vi "AlliGator Run Source Image Python Function.vi"(8 "error in (no error)":errorcluster, 9 "Source Image":T5, 10 "Python Function Info":T1={"Script Path"=path "", "Function Name"="", "Function Parent Menu"="", "Function Input Parameters"=[], "Function Outputs"=[], "Function Doc String"="", "Function Display Name"="", "Function Target Type"=enum."Window Menu", "Function Target Window"="", "Parent Menu Location"="", "Item Menu Tag"="", "Is preceded by Separator"=FALSE}, 11 "Data Value Reference in":refnum<data-value>) -> (0 "error out":errorcluster, 1 "Message":string, 2 "Function Output Type":string, 3 "Data Value Reference out":refnum<data-value>)   [LabVIEW 2021, in "AlliGator Python Plugins.lvlib"]
doc: "Runs image-related python function."
uses:
  AlliGator Python Plugins.lvlib
  AlliGator Internal Variables v2.ctl
  <vilib>/vision/Image Controls.llb/IMAQ Image.ctl
  AlliGator Gate Image Set.ctl
  AlliGator FLI Dataset Type.ctl
  AlliGator Data Series Type.ctl
  AlliGator Dataset Channel.ctl
  AlliGator Gate Arithmetic.ctl
  AlliGator Displayed Image.ctl
  Image/Named ROI Description.ctl
  AlliGator Decay Metadata v3.ctl
  AlliGator Decay Background Subtraction Info.ctl
  AlliGator Baseline Subtraction Method.ctl
  Graphs/XY Graph/XY Graph Plot Shift Parameters.ctl
  Graphs/XY Graph/XY Graph Plot Shift Method.ctl
  AlliGator Decay Extrapolation Parameters.ctl
  Phasor/Calibration Phasor (m, phi).ctl
  Phasor/Phasor Reference Series.ctl
  Phasor/Phasor Calibration Map v2.ctl
  Phasor/Phasor (g, s).ctl
  AlliGator Raw Phasor Plot Data v4.ctl
  Phasor/Phasor Standard Deviation Options.ctl
  AlliGator Phasor Multi-Harmonic Data.ctl
  Phasor/Phasor Harmonic Data.ctl
  AlliGator Decay Fit Options & Parameters v2.ctl
  Fits/IRF(X)PSED/Decay Fit Options v2.ctl
  Fits/Decay Convolution/Decay Model.ctl
  Fits/Residual Type.ctl
  Fits/IRF(X)PSED/Fit Weights Type.ctl
  Fits/Non-linear Fitting Method v2.ctl
  Fits/Fit Calculation Method.ctl
  Fits/Non-linear Fitting Algorithm.ctl
  AlliGator Decay Fit Parameter Constraints 2.ctl
  Fits/IRF(X)PSED/Decay Fit Parameters In List.ctl
  Fits/IRF(X)PSED/MLE Baseline Offset Type.ctl
  AlliGator Decay Preprocessing Parameters.ctl
  Fits/IRF(X)PSED/Decay Fit Parameters & Derived Quantities List.ctl
  AlliGator Python Function Information.ctl
  AlliGator Python Function Parameter Definition.ctl
  AlliGator Python Function Output Definition.ctl
  AlliGator Python Plugin Target Type.ctl
  AlliGator Variables List.ctl
  AlliGator Python Plugin Image Data.ctl
  AlliGator Globals, Variables & Constants.lvlib
  AlliGator Source Image.lvlib
  Error/Error.lvlib
  Phasor/Phasor.lvlib
  Image/Image.lvlib
  AlliGator Decay Preprocessing.lvlib
  Graphs/XY Graph/XY Graph Add-Ons.lvlib
  AlliGator Phasor Graph.lvlib
  AlliGator Files.lvlib
  AlliGator Phasor Plot.lvlib
  Fits/Fits.lvlib
  AlliGator Decay Fit.lvlib
  AlliGator Decay Fit Parameter Map.lvlib
  AlliGator Internal Variables.lvlib
  AlliGator Settings.lvlib
  AlliGator Dual-Channel Datasets.lvlib
panel:
  out "session out":refnum<k35>
  out "Function Parameters String":string
  # "see the AlliGator License on the block diagram (Ctrl+E or Window:Show Block Diagram)"
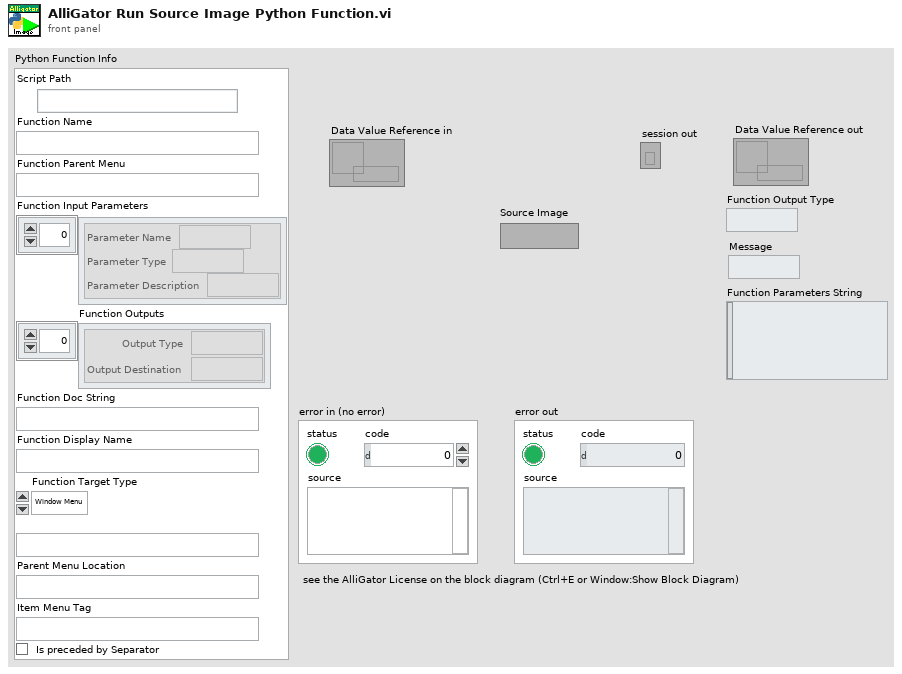
[diagram p1: front panel]
types:
  T1 = typedef "AlliGator Python Plugins.lvlib/AlliGator Python Function Information.ctl" = cluster{"Script Path":path, "Function Name":string, "Function Parent Menu":string, "Function Input Parameters":T2[], "Function Outputs":T3[], "Function Doc String":string, "Function Display Name":string, "Function Target Type":T4, "Function Target Window":string, "Parent Menu Location":string, "Item Menu Tag":string, "Is preceded by Separator":bool}
  T2 = typedef "AlliGator Python Plugins.lvlib/AlliGator Python Function Parameter Definition.ctl" = cluster{"Parameter Name":string, "Parameter Type":string, "Parameter Description":string}
  T3 = typedef "AlliGator Python Plugins.lvlib/AlliGator Python Function Output Definition.ctl" = cluster{"Output Type":string, "Output Destination":string}
  T4 = typedef "AlliGator Python Plugins.lvlib/AlliGator Python Plugin Target Type.ctl" = enum16{"Undefined", "Window Menu", "Object Menu"}
  T5 = typedef "IMAQ Image.ctl" = refnum<image>
  T6 = typedef "AlliGator Python Plugins.lvlib/AlliGator Python Plugin Image Data.ctl" = cluster{"Image_Name":string, "Image":sgl[][]}
  T7 = typedef "AlliGator Source Image.lvlib/AlliGator Displayed Image.ctl" = enum16{"Single Gate", "Sum of All Gates", "Max of All Gates", "Min of All Gates", "-", "White Ligth Image", "Mask Image"}
  T8 = typedef "AlliGator Globals, Variables & Constants.lvlib/AlliGator Variables List.ctl" = enum16{"---- GUI ----", "Initialization Status", "State Indicators Refnum", "Original AlliGator Menu Items", "Current Action Loop State", "Script in progress", "Playback", "Loop Playback", "Search ROI Used", "Search ROI", "Decay Graph Max Legend Size", "Intensity Graph Max Legend Size", "Decay Statistics Graph Max Legend Size", "Phasor Graph Max Legend Size", "Phasor Ratio Graph Max Legend Size", "Lifetime Graph Max Legend Size", "---- Files ----", "Export Dataset Frames as Individual Files", "Show Batch Export Help Balloons", "Frames in Dataset", "ptu File Frame Start Indices", "Current Frame in Dataset", "Current Frame Timestamp", "------ Python Plugins ------", "Python Plugins Information", "Python Session", "Valid Python Session?", "---- Source Image ----", "Dataset Loaded", "Dataset Metadata", "Dataset Channel", "Dataset Data Description", "Background Dataset Metadata", "Background Dataset Channel", "Background Dataset Data Description", "Background File Subtraction", "Background File Path", "Background File Pile-up Correction", "Background File Pixel Well Capacity", "Background File Scaling Factor", "Source Image ROIs", "Current Source Image ROI", "Source Image ROI Event Refnum", "X_Source Image Display Range", "X_Source Image Palette Information", "Source Image Palette List", "Source Image Scale", "Current Dataset Load Settings", "Source Image:ROI Overlay Color", "---- Image Profile Window ----", "Image Profile:Overlay ROI in Source Image", "Image Profile Window Event Refnum", "Image Profile:IntensityType", "Image Profile:Intensity Average Type", "Image Profile:Intensity-weighted SDV", "Image Profile:Box Profile Type", "Image Profile Window Open", "Image Profile:Plotted Fit Parameter", "X_Type of Displayed Image", "X_Time Gate Slider", "Dataset Path", "Source Image Overlay to Erase", "Is Displayed Image Accumulated", "White Light Image Modified", "Mask Image Modified", "Macrotime Gate Separation", "------ Phasor Graph -------", "Phasor Graph:Show Line", "---- Phasor Plot ---", "Phasor Plot Parameters Changed", "FLI Dataset Modified since last Phasor Plot Calculation", "Phasor Harmonics Data", "Selected Phasor Harmonics", "Phasor Harmonic Manager Event Refnum", "Phasor Plot ROIs", "Current Phasor Plot ROI", "Phasor Plot ROI Event Refnum", "Phasor Plot Image Reference Points", "Phasor Plot Computed", "Phasor Plot Palette Information", "Phasor Plot Palette List", "Phasor Ratio Palette Information", "Phasor Ratio Palette List", "Phasor Image Scale", "Phasor Plot Image Overlay to Erase", "Phasor Plot Image Elements to Update", "Current Phasor Plot Calculation Parameters", "Current Phasor Calibration Options", "Reset Cumulated Phasor Plot", "Phasor Ratio Reference 1", "Phasor Ratio Lifetime Reference 1", "Phasor Ratio Reference 1 Frequency", "Phasor Ratio Reference 2", "Phasor Ratio Lifetime Reference 2", "Phasor Ratio Reference 2 Frequency", "---- Decay Analysis ----", "Number of Selected Decays to Fit", "LS Fit Results", "LAR Fit Results", "BS Fit Results", "Last Decay Max - Min", "Best Fit Parameters", "Best Fit Parameter Names", "Actual Size X", "Actual Size Y", "Binning X", "Binning Y", "Actual # Gates", "Dataset Number", "Gates to...", "Gates Skipped", "Gates to keep", "Gate Step", "Gate Separation", "Reversed Gates", "Pile-up Correction", "Pixel Well Capacity", "Background Subtracted", "Background Subtraction Method", "Background Definition Range", "Background File (deprecated)", "Number of Dataset Accumulated", "Array of Accumulated Dataset Paths", "Do Averaged Datasets", "Destination File Path", "Process Plot Target", "Use 1/D as Phasor Frequency", "---- Decay Fit Parameter Map -----", "Decay Fit Parameter Map Palette Information", "Decay Fit Parameter Map Palette List", "Local Decay Graph Window Event Refnum", "------- Local Decay Window ---------", "Use normalized IRF for convolution", "----- Miscellaneous ----", "Skippable Dialog Windows Status"}
  T9 = typedef "AlliGator Internal Variables.lvlib/AlliGator Internal Variables v2.ctl" = cluster{"Displayed Image":T5, "White Light Image":T5, "Mask Image":T5, "ROI Mask Image":T5, "Current Dataset Images 1":T10, "Background Dataset Images 1":T10, "Current Dataset Images 2":T10, "Background Dataset Images 2":T10, "Current Dataset Arithmetic Images":T10, "Accumulated Dataset Images 1":T10, "Accumulated Dataset Images 2":T10, "Accumulated Dataset Arithmetic Images":T10, "Phasor Plot Image":T5, "Decay Fit Parameter Map Image":T5, "Single Data Point Path":path, "White Light Image Path":path, "Mask Image Path":path, "Time-Series Folder":path, "[Time-Series Paths]":path[], "Current Dataset":i32, "Single Dataset Type":T11, "Current Folder":string, "AlliGator Data Series Type":T12, "# Datasets":i32, "Dual-Channel Dataset":bool, "Selected Channel Name":string, "Dataset Channel":T13, "Channel Arithmetic":T14, "Dual-Channel Background Dataset":bool, "Background Channel":T13, "Dual-Channel Accumulated Dataset":bool, "Start Time":dbl, "[Time-Series Timestamps]":dbl[], "[Intensity Corrections]":dbl[], "Time Series Script":bool, "Type of Displayed Image":T7, "Gate Image Slide":u16, "# Gates":i32, "ROIs":T15[], "ROI Decay":cluster{"t Array":dbl[], "I Array":dbl[]}, "Valid Decay":bool, "Decay  Metadata":T17, "Reference Decay Plot Name":string, "Reference Decay":cluster{"t Array":dbl[], "I Array":dbl[]}, "Decay Shift Plot":cluster{"Time Stamps":dbl[], "Decay Shifts":dbl[]}, "[Decays Max Values]":sgl[], "[Decays Min Values]":sgl[], "Calibration Phasor":T23, "Calibration Phasor Series":T24, "Phasor Calibration Map":T25, "Calibration Map MD5 Digest":string, "Last Raw Phasor":T26, "Last Calibrated Phasor":T26, "Last Calibrated Phasor SDV":T26, "Phasor Graph:Phasor Plot":cluster{"g Array":dbl[], "s Array":dbl[]}, "Phasor Graph:Phasor SDV Plot":cluster{"g Array":dbl[], "s Array":dbl[]}, "[Phasor Graph:Raw Phasor Plots]":T27[], "Phasor Plot locked to Ref 1":i32, "[Phasor Plot(s) locked to Ref 1]":i32[], "[Phasor Plot(s) locked to Ref 2]":i32[], "[Pixel Phasors]":T26[], "[[Sum Image]]":dbl[][], "[[CSG Phasors]]":csg[][], "[[Valid Pixel?]]":bool[][], "I/m/phi Dataset":cluster{"I/m/phi Dataset?":bool, "Base Frequency":dbl[unit], "Harmonic Orders":u8[]}, "Multi Phasor Plot Data":T29, "Decay Fit Options & Parameters":T31, "Fit Options: Decay Preprocessing Parameters":T42, "Fit Options: Reference Decay":cluster{"t Array":dbl[], "I Array":dbl[]}, "Is Full Image Parameters Map":bool, "Is Single-Pixels Parameters Map":bool, "NLSF Parameters Map X Resolution":i32, "NLSF Parameters Map Y Resolution":i32, "[Single Decay Fit Parameters]":dbl[], "Fit Model":T33, "[[Multiple Decays Fit Parameters]]":dbl[][], "[[Multiple Decays Fit Parameter SDVs]]":dbl[][], "[[IRFs]]":dbl[][], "IRF Array Time Axis":dbl[], "Decay Array Time Axis":dbl[], "[Decay Fit Parameter Names]":T43[], "[[Phasor Ratios]]":dbl[][], "[[Average Lifetimes]]":dbl[][], "Amplitude Weighted Average Lifetime":bool, "[Decay Sum]":dbl[], "[[User-defined Quantities]]":dbl[][], "User-defined Quantity":string}
  T10 = typedef "AlliGator Internal Variables.lvlib/AlliGator Gate Image Set.ctl" = cluster{"SGL Image Max":T5, "SGL Image Sum":T5, "SGL Gate Images":T5[], "SGL Image Min":T5}
  T11 = typedef "AlliGator Files.lvlib/AlliGator FLI Dataset Type.ctl" = enum16{"HDF5 FLI Dataset", "Gate Image Folder", ".sdt FLI Dataset (Becker & Hickl)", ".ptu FLI Dataset (PicoQuant)", "SS1 FLI Dataset", "SS2 FLI Dataset", "I/m/phi Dataset", ".bin FLI Dataset (PicoQuant Binned)", ".bin FLI Dataset (Piccolo Binned)"}
  T12 = typedef "AlliGator Files.lvlib/AlliGator Data Series Type.ctl" = enum16{"Not a Supported Series", "Gate Images Folder Series", "SwissSPAD 2 Dataset Series", "B&H FLI Dataset Series", "PicoQuant PTU FLI Dataset Series", "PicoQuant BIN FLI Dataset Series", "Piccolo hist BIN FLI Dataset Series", "HDF5 FLI Dataset Series"}
  T13 = typedef "AlliGator Dual-Channel Datasets.lvlib/AlliGator Dataset Channel.ctl" = enum16{"G2", "INT"}
  T14 = typedef "AlliGator Settings.lvlib/AlliGator Gate Arithmetic.ctl" = enum16{"None", "INT-G2", "G2/INT*<INT>", "(1 - G2/INT)*<INT>"}
  T15 = typedef "Image.lvlib/Named ROI Description.ctl" = cluster{"ROI Descriptor":T16, "ROI Name":string, "Overlay Color":u32}
  T16 = typedef "ROI Descriptor" = cluster{"Global Rectangle":i32[], "Contours":cluster{"ID":enum32{"External", "Internal"}, "Type":u32, "Coordinates":i32[]}[]}
  T17 = typedef "AlliGator Phasor Graph.lvlib/AlliGator Decay Metadata v3.ctl" = cluster{"ROI Descriptor":T16, "ROI Center":cluster{"X":i32, "Y":i32}, "Decay Background Subtraction Info":T18, "Decay Reverted":bool, "Decay Smoothened":bool, "Decay Straightened":bool, "Fitted Tau (Decay Straightening)":dbl, "Decay Shift Parameters":T20, "Decay Shifted":bool, "Decay Extrapolated":bool, "Decay Extrapolation Parameters":T22, "Decay Normalized":bool, "Fold Decay":bool, "# Folds":u32}
  T18 = typedef "AlliGator Decay Analysis.lvlib/AlliGator Decay Preprocessing.lvlib/AlliGator Decay Background Subtraction Info.ctl" = cluster{"Laser Period":dbl[unit], "Gate Duration":dbl[unit], "Baseline Subtraction Method":T19, "Background Definition Range":cluster{"Min Gate":dbl[unit], "Max Gate":dbl[unit]}, "Total Intensity w/o Bkgd Subtraction":dbl, "Bkgd-subtracted Intensity (exp)":dbl, "# Data Points":i32, "Background/Gate":dbl, "Fitted Lifetime":dbl[unit], "Bkgd-subtracted Intensity (theo)":dbl}
  T19 = typedef "AlliGator Decay Analysis.lvlib/AlliGator Decay Preprocessing.lvlib/AlliGator Baseline Subtraction Method.ctl" = enum16{"Mean", "Min", "Square Gated Single-Exponential", "File", "Constant"}
  T20 = typedef "XY Graph Add-Ons.lvlib/XY Graph Plot Shift Parameters.ctl" = cluster{"Type":T21, "Shift":dbl[unit], "Threshold":dbl, "Rotate":bool}
  T21 = typedef "XY Graph Add-Ons.lvlib/XY Graph Plot Shift Method.ctl" = enum16{"Default", "CFD", "Threshold", "Cross-Correlation"}
  T22 = typedef "AlliGator Decay Analysis.lvlib/AlliGator Decay Preprocessing.lvlib/AlliGator Decay Extrapolation Parameters.ctl" = cluster{"Additional Points":u32, "Head Fraction":dbl, "Fitted Tau":dbl, "Use Periodicity":bool, "Use Cursors":bool, "Tail Fraction":dbl}
  T23 = typedef "Phasor.lvlib/Calibration Phasor (m, phi).ctl" = cluster{"m":dbl, "phi":dbl, "Phasor Frequency":dbl[unit], "Reference Lifetime":dbl[unit]}
  T24 = typedef "Phasor.lvlib/Phasor Reference Series.ctl" = cluster{"m Array":dbl[], "phi Array":dbl[], "Phasor Frequency":dbl[unit], "Calibration Lifetime":dbl[unit]}
  T25 = typedef "Phasor.lvlib/Phasor Calibration Map v2.ctl" = cluster{"Phasor Frequency":dbl[unit], "Calibration Lifetime":dbl[unit], "ROI Centers":cluster{"X":i32, "Y":i32}[], "ROI Descriptors":T16[], "Map Resolution X":i32, "Map Resolution Y":i32, "z Array":cdb[]}
  T26 = typedef "Phasor.lvlib/Phasor (g, s).ctl" = cluster{"g":dbl, "s":dbl}
  T27 = typedef "AlliGator Phasor Graph.lvlib/AlliGator Raw Phasor Plot Data v4.ctl" = cluster{"Phasor Plot Name":string, "Raw Phasor Plot":T26[], "Phasor Frequency":dbl[unit], "[Decay Metadata]":T17[], "Raw Phasor Plot SDV":T26[], "Phasor SDV Options":T28, "[Calibration Phasor]":T23[]}
  T28 = typedef "Phasor.lvlib/Phasor Standard Deviation Options.ctl" = cluster{"Compute Estimated SDV":bool, "# Replicas":u32, "Use Estimated Average Phasor":bool}
  T29 = typedef "AlliGator Phasor Plot.lvlib/AlliGator Phasor Multi-Harmonic Data.ctl" = cluster{"Base Frequency":dbl[unit], "# Harmonics":u8, "Harmonic Orders":u8[], "Phasor Plot Settings Checksum":u64, "Phasor Harmonic Data Array":T30[]}
  T30 = typedef "Phasor.lvlib/Phasor Harmonic Data.ctl" = cluster{"Phasor Harmonic Name":string, "Phasor Plot Settings Checksum":u64, "Phasor Frequency":dbl[unit], "Base Frequency":dbl[unit], "Harmonic Order":u8, "Phasor Plot Parameters":string, "Phasor Array [[CSG]]":csg[][], "Dataset File Path":path}
  T31 = typedef "AlliGator Decay Fit Parameter Map.lvlib/AlliGator Decay Fit Options & Parameters v2.ctl" = cluster{"SYNC Period":dbl[unit], "Fit Options":T32, "Fit Parameter Constraints":T39[], "MLE Baseline Offset":dbl, "MLE Baseline Offset Type":T41}
  T32 = typedef "Fits.lvlib/Decay Fit Options v2.ctl" = cluster{"Show Fit Residuals":bool, "Fit Model":T33, "Residual Type":T34, "Max Decay Percentile":dbl, "Min Decay Percentile":dbl, "Show Full Decay":bool, "Weights":T35, "Fitting Method":T36, "Compute Parameter Uncertainties":bool, "Periodic Boundaries":bool, "Model Calculation":T37, "Period":dbl[unit], "Termination Criteria":cluster{"Max Iterations":i32, "Max Function Calls":i32, "Max Time":dbl[unit], "Function Tolerance":dbl, "Parameter Tolerance":dbl, "Gradient Tolerance":dbl, "Min Lambda":dbl, "Max Lambda":dbl, "Initial Tick Count":u32}, "Offset Resolution":dbl[unit], "Use Local IRF":bool, "Fitting Algorithm":T38}
  T33 = typedef "Fits.lvlib/Decay Model.ctl" = enum16{"1-Exponential", "2-Exponentials"}
  T34 = typedef "Fits.lvlib/Residual Type.ctl" = enum16{"Standard", "Normalized", "Reduced"}
  T35 = typedef "Fits.lvlib/Fit Weights Type.ctl" = enum16{"Unweighted", "1/Variance", "Best of All"}
  T36 = typedef "Fits.lvlib/Non-linear Fitting Method v2.ctl" = enum16{"Least Square", "Least Absolute Residual", "Bisquare", "MLE", "-", "Best of All"}
  T37 = typedef "Fits.lvlib/Fit Calculation Method.ctl" = enum16{"Simulation", "Convolution", "Integration"}
  T38 = typedef "Fits.lvlib/Non-linear Fitting Algorithm.ctl" = enum16{"Levenberg-Marquardt", "Trust-Region Dogleg"}
  T39 = typedef "AlliGator Decay Analysis.lvlib/AlliGator Decay Fit.lvlib/AlliGator Decay Fit Parameter Constraints 2.ctl" = cluster{"Fit Parameter":T40, "Min Value":dbl, "Max Value":dbl, "Global":bool, "Used":bool}
  T40 = typedef "Fits.lvlib/Decay Fit Parameters In List.ctl" = enum16{"Offset", "Baseline", "A_1", "tau_1", "A_2", "tau_2"}
  T41 = typedef "Fits.lvlib/MLE Baseline Offset Type.ctl" = enum32{"Absolute", "Percentage"}
  T42 = typedef "AlliGator Decay Analysis.lvlib/AlliGator Decay Preprocessing.lvlib/AlliGator Decay Preprocessing Parameters.ctl" = cluster{"Background Subtraction":bool, "Straighten Decay":bool, "Reverse Gates":bool, "1-Normalized Decay":bool, "Smoothen Decay":bool, "Smoothing Parameter":dbl, "Shift Decay":bool, "Decay Shift Parameters":T20, "Extrapolate Decay":bool, "Additional Points":u32, "Head Fraction":dbl, "Pixel-Normalize Decay":bool, "Use Periodicity":bool, "Use Cursors":bool, "Tail Fraction":dbl, "Use Decay Pre-Processing":bool, "Fold Decay":bool, "# Folds":u32, "[0-1]-Normalized Decay":bool}
  T43 = typedef "Fits.lvlib/Decay Fit Parameters & Derived Quantities List.ctl" = enum16{"Offset", "Baseline", "A_1", "tau_1", "A_2", "tau_2", "<tau>_a", "f1_a", "f2_a", "<tau>_i", "f1_i", "f2_i", "-", "R^2", "Chi^2"}
  T44 = typedef "Image Type" = u32
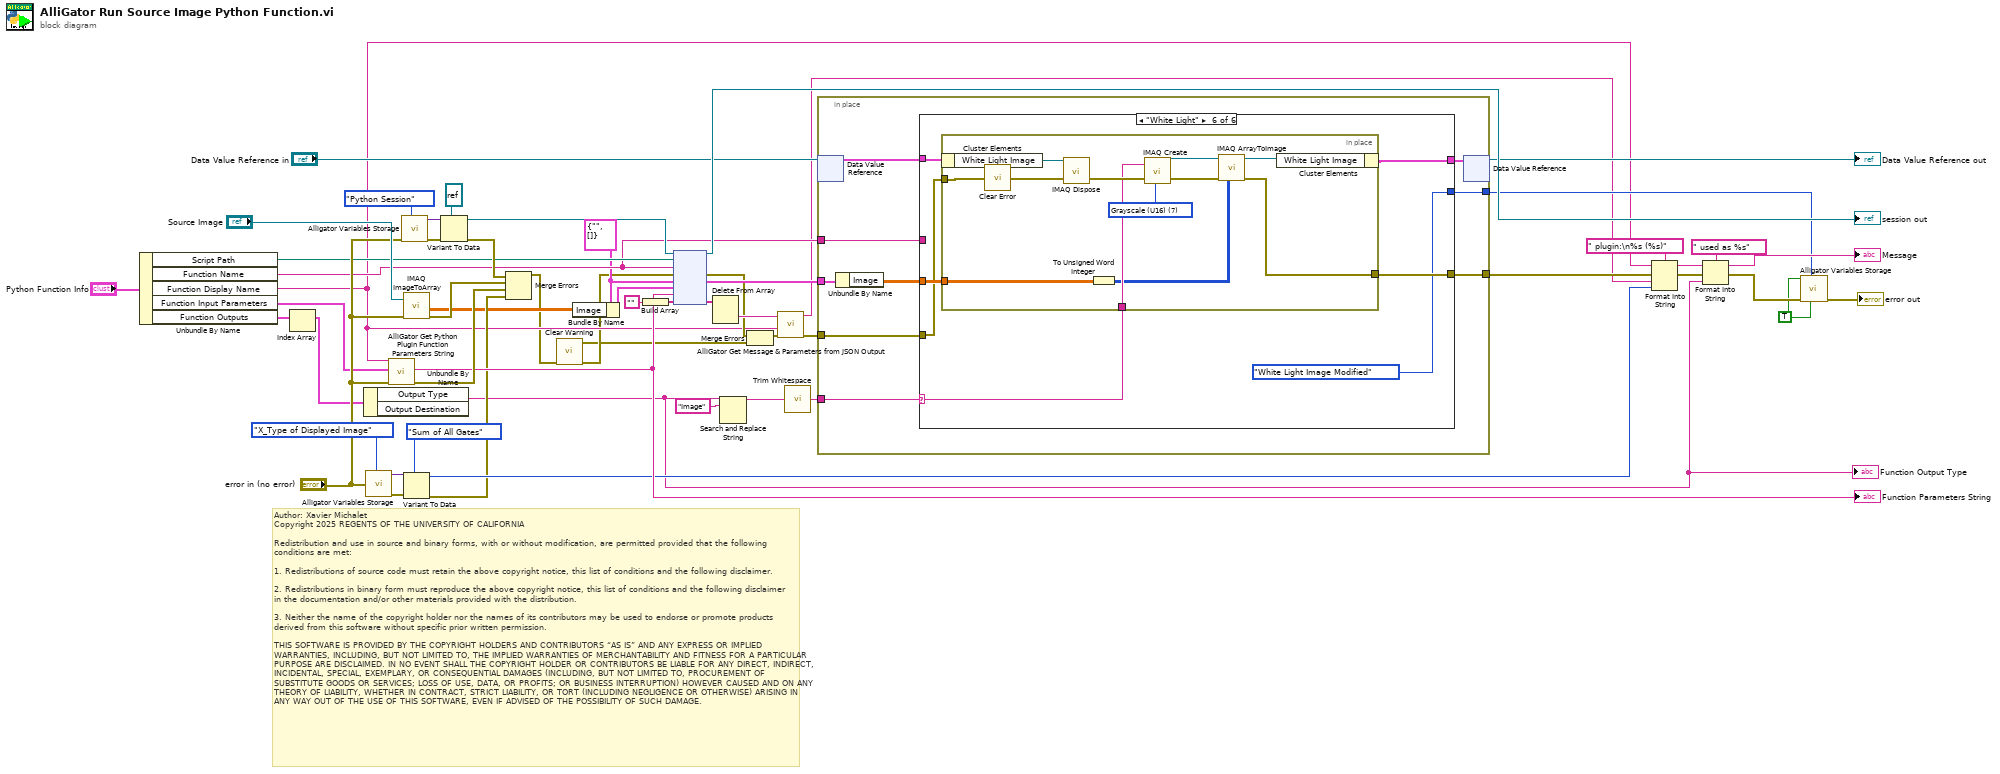
[diagram p0: block diagram]
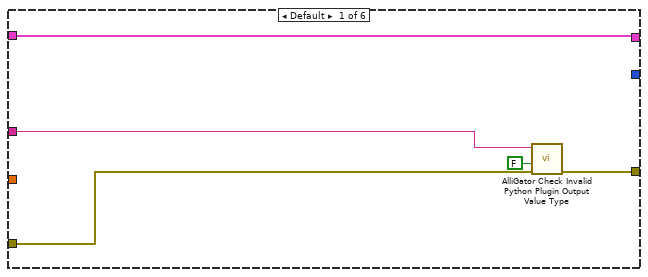
[diagram p2: hidden frame]
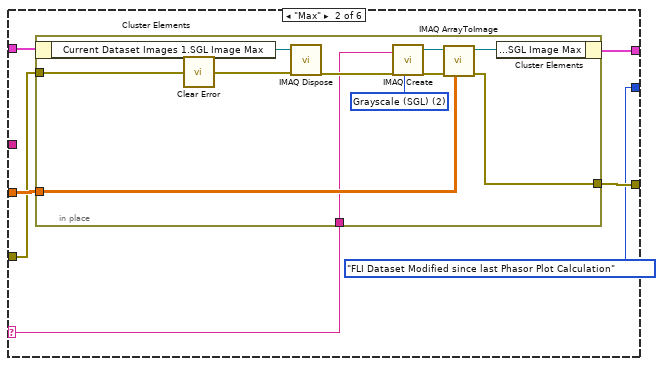
[diagram p3: hidden frame]
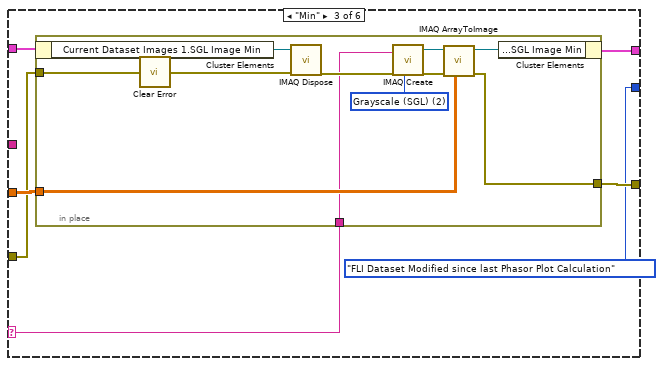
[diagram p4: hidden frame]
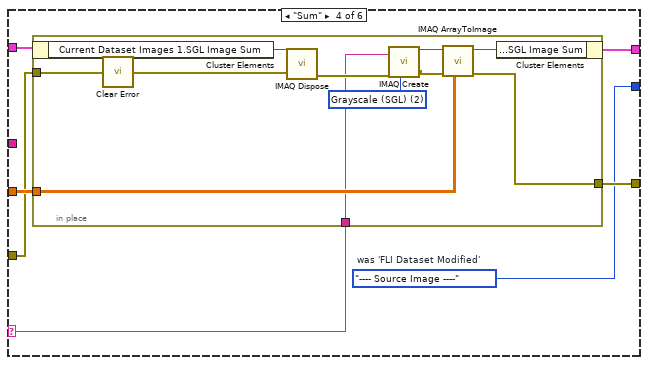
[diagram p5: hidden frame]
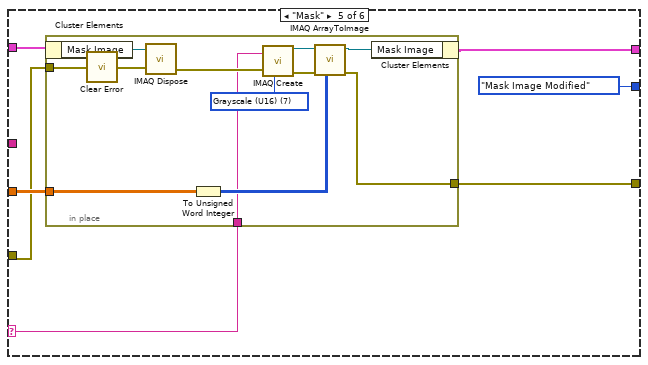
[diagram p6: hidden frame]
diagram:
  w9 = T6 {"Image_Name"="", "Image"=[]} ("Image_Data")
  w32 = TRUE ("Get(F)/Set")
  # "Author: Xavier Michalet\nCopyright 2025 REGENTS OF THE UNIVERSITY OF CALIFORNIA\n\nRedistribution and use in source and binary forms, with or without modification, are permitted provided that the following conditions are met:\n\n1. Redistributions of source code must retain the above copyright notice, this list of conditions and the following disclaimer.\n\n2. Redistributions in binary form must reproduce the above copyright notice, this list of conditions and the following disclaimer in the documentation and/or other materials provided with the distribution.\n\n3. Neither the name of the copyright holder nor the names of its contributors may be used to endorse or promote products derived from this software without specific prior written permission.\n\nTHIS SOFTWARE IS PROVIDED BY THE COPYRIGHT HOLDERS AND CONTRIBUTORS “AS IS” AND ANY EXPRESS OR IMPLIED WARRANTIES, INCLUDING, BUT NOT LIMITED TO, THE IMPLIED WARRANTIES OF MERCHANTABILITY AND FITNESS FOR A PARTICULAR PURPOSE ARE DISCLAIMED. IN NO EVENT SHALL THE COPYRIGHT HOLDER OR CONTRIBUTORS BE LIABLE FOR ANY DIRECT, INDIRECT, INCIDENTAL, SPECIAL, EXEMPLARY, OR CONSEQUENTIAL DAMAGES (INCLUDING, BUT NOT LIMITED TO, PROCUREMENT OF SUBSTITUTE GOODS OR SERVICES; LOSS OF USE, DATA, OR PROFITS; OR BUSINESS INTERRUPTION) HOWEVER CAUSED AND ON ANY THEORY OF LIABILITY, WHETHER IN CONTRACT, STRICT LIABILITY, OR TORT (INCLUDING NEGLIGENCE OR OTHERWISE) ARISING IN ANY WAY OUT OF THE USE OF THIS SOFTWARE, EVEN IF ADVISED OF THE POSSIBILITY OF SUCH DAMAGE."
  n1 = Unbundle By Name("Python Function Info") -> ("Script Path"=w27:path, "Function Name"=w16:string, "Function Display Name"=w5:string, "Function Input Parameters"=w26:T2[], "Function Outputs"=w22:T3[])
  n2 = Index Array(array=w22) -> (element=w20:T3)  [unwired: 1 in]
  n3 = Unbundle By Name(w20) -> ("Output Type"=w19:string)  [unwired: 1 out]
  "Function Output Type" <- w19
  n4 = call "Alligator Variables Storage.vi"("AlliGator Variable"=AlliGator_Variables_List."X_Type of Displayed Image" ("Alligator Variable"), "Error In"="error in (no error)") -> ("Error Out"=w41:errorcluster, "Data out"=w42:variant)  [unwired: 7 in, 1 out]
  n5 = call "AlliGator Get Python Plugin Function Parameters String.vi"("error in (no error)"="error in (no error)", "Function Parameters"=w26, "Function Display Name"=w5) -> ("error out"=w54:errorcluster, "Function Parameters JSON String"=w53:string)  [unwired: 6 in, 1 out]
  "Function Parameters String" <- w53
  n6 = call "Alligator Variables Storage.vi"("AlliGator Variable"=AlliGator_Variables_List."Python Session" ("Alligator Variable"), "Error In"="error in (no error)") -> ("Error Out"=w51:errorcluster, "Data out"=w49:variant)  [unwired: 7 in, 1 out]
  n7 = call "IMAQ ImageToArray"("error in (no error)"="error in (no error)", "Image"="Source Image") -> ("Image Pixels (Float)"=w7:sgl[][], "error out"=w29:errorcluster)  [unwired: 2 in, 3 out]
  n8 = Variant To Data(error in=w41, type=AlliGator_Displayed_Image."Sum of All Gates" ("Displayed Image"), Variant=w42) -> (data=w39:T7, error out=w38:errorcluster)
  n9 = Variant To Data(error in=w51, type=refnum<k35> refnum ("session in"), Variant=w49) -> (data=w47:refnum<k35>, error out=w50:errorcluster)
  n10 = Merge Errors(w50, w29, w54, w38) -> (w4:errorcluster)
  n11 = call "Clear Warning.vi"("error in (no error)"=w4) -> ("cleared warning or error dup"=w3:errorcluster, "error in (dup)"=w1:errorcluster)  [unwired: 9 in]
  n12 = Bundle By Name(cluster=w9, "Image"=w7) -> (w8:T6)
  n13 = Build Array("") -> (w15:string[])
  n14 = node(w47, w27, w16, w3, w9, w8, w53, w15) -> (→"session out":refnum<k35>, w11:errorcluster, w25:T6, w12:string[])  [unwired: 2 in, 2 out]
  n15 = Delete From Array(array=w12) -> (deleted portion=w13:string)  [unwired: 2 in, 1 out]
  n16 = Search and Replace String(input string=w19, search string="Image") -> (result string=w23:string)  [unwired: 6 in, 3 out]
  n17 = Merge Errors(w11, w1) -> (w2:errorcluster)
  n18 = call "AlliGator Get Message & Parameters from JSON Output.vi"("error in (no error)"=w2, "Function Display Name"=w5, "<JSON>"=w13) -> ("error out"=w10:errorcluster, "Notebook Message"=w6:string)  [unwired: 7 in]
  n19 = call <vilib>:"Trim Whitespace.vi"("string"=w23) -> ("trimmed string"=w21:string)  [unwired: 1 in]
  n20 = in-place {
    in-place-border: [w65] -> w56
    in-place-border: [w64] -> w33
    in-place-border: w25 -> [w63]
    in-place-border: w21 -> [w62]
    in-place-border: w16 -> [w58]
    in-place-border: w10 -> [w57]
    n21 = in-place-dvr #1("Data Value Reference in") -> (w60:T9)  [unwired: 1 out]
    n22 = Unbundle By Name(w63) -> ("Image"=w61:sgl[][])
    n23 = case shown="\"White Light\"" w62 {
      selector: w62 -> [_ w74 w92 w110 w128 w148]
      tunnel: w61 -> [_ w77 w95 w113 w131 w150]
      tunnel: [w69 w76 w94 w112 w130 w149] -> w65
      tunnel: [_ AlliGator_Variables_List."FLI Dataset Modified since last Phasor Plot Calculation" ("Alligator Variable") AlliGator_Variables_List."FLI Dataset Modified since last Phasor Plot Calculation" ("Alligator Variable") w111 AlliGator_Variables_List."Mask Image Modified" ("Alligator Variable") AlliGator_Variables_List."White Light Image Modified" ("Alligator Variable")] -> w64
      tunnel: w60 -> [w70 w73 w91 w109 w127 w146]
      tunnel: [w70 w72 w90 w108 w126 w145] -> w59
      tunnel: w58 -> [w68 _ _ _ _ _]
      tunnel: w57 -> [w66 w71 w89 w107 w125 w144]
      frame Default {
        n24 = call "AlliGator Check Invalid Python Plugin Output Value Type.vi"("error in (no error)"=w66, "Valid Output Value Type?"=FALSE, "Source"=w68) -> ("error out"=w69:errorcluster)  [unwired: 8 in]
      }
      frame "Max" {
        n25 = in-place {
          in-place-border: w77 -> [w87]
          in-place-border: w71 -> [w84]
          in-place-border: [w86] -> w76
          in-place-border: w74 -> [w79]
          w80 = T44 2 items=["Grayscale (U8)", "Grayscale (I16)", "Grayscale (SGL)", "Complex (CSG)", "RGB (U32)", "HSL (U32)", "RGB (U64)", "Grayscale (U16)"] ("Image Type")
          n26 = in-place-cluster #2(w73) -> ("Current Dataset Images 1.SGL Image Max"=w85:T5)
          n27 = call "Clear Error.vi"("Error In"=w84) -> ("no Error Out"=w78:errorcluster)  [unwired: 8 in]
          n28 = call "IMAQ Dispose"("Image"=w85, "error in (no error)"=w78) -> ("error out"=w83:errorcluster)  [unwired: 4 in]
          n29 = call "IMAQ Create"("Image Name"=w79, "Image Type"=w80, "error in (no error)"=w83) -> ("New Image"=w81:T5, "error out"=w82:errorcluster)  [unwired: 2 in]
          n30 = call "IMAQ ArrayToImage"("Image Pixels (Float)"=w87, "error in (no error)"=w82, "Image"=w81) -> ("error out"=w86:errorcluster, "Image Out"=w88:T5)  [unwired: 7 in]
          n31 = in-place-cluster #2("Current Dataset Images 1.SGL Image Max"=w88) -> (w72:T9)
        }
      }
      frame "Min" {
        n32 = in-place {
          in-place-border: w95 -> [w105]
          in-place-border: w89 -> [w102]
          in-place-border: [w104] -> w94
          in-place-border: w92 -> [w97]
          w98 = T44 2 items=["Grayscale (U8)", "Grayscale (I16)", "Grayscale (SGL)", "Complex (CSG)", "RGB (U32)", "HSL (U32)", "RGB (U64)", "Grayscale (U16)"] ("Image Type")
          n33 = in-place-cluster #3(w91) -> ("Current Dataset Images 1.SGL Image Min"=w103:T5)
          n34 = call "Clear Error.vi"("Error In"=w102) -> ("no Error Out"=w96:errorcluster)  [unwired: 8 in]
          n35 = call "IMAQ Dispose"("Image"=w103, "error in (no error)"=w96) -> ("error out"=w101:errorcluster)  [unwired: 4 in]
          n36 = call "IMAQ Create"("Image Name"=w97, "Image Type"=w98, "error in (no error)"=w101) -> ("New Image"=w99:T5, "error out"=w100:errorcluster)  [unwired: 2 in]
          n37 = call "IMAQ ArrayToImage"("Image Pixels (Float)"=w105, "error in (no error)"=w100, "Image"=w99) -> ("error out"=w104:errorcluster, "Image Out"=w106:T5)  [unwired: 7 in]
          n38 = in-place-cluster #3("Current Dataset Images 1.SGL Image Min"=w106) -> (w90:T9)
        }
      }
      frame "Sum" {
        w111 = AlliGator_Variables_List."---- Source Image ----"  # was 'FLI Dataset Modified'
        n39 = in-place {
          in-place-border: w113 -> [w123]
          in-place-border: [w122] -> w112
          in-place-border: w110 -> [w116]
          in-place-border: w107 -> [w115]
          w120 = T44 2 items=["Grayscale (U8)", "Grayscale (I16)", "Grayscale (SGL)", "Complex (CSG)", "RGB (U32)", "HSL (U32)", "RGB (U64)", "Grayscale (U16)"] ("Image Type")
          n40 = in-place-cluster #4(w109) -> ("Current Dataset Images 1.SGL Image Sum"=w119:T5)
          n41 = call "Clear Error.vi"("Error In"=w115) -> ("no Error Out"=w114:errorcluster)  [unwired: 8 in]
          n42 = call "IMAQ Dispose"("Image"=w119, "error in (no error)"=w114) -> ("error out"=w121:errorcluster)  [unwired: 4 in]
          n43 = call "IMAQ Create"("Image Name"=w116, "Image Type"=w120, "error in (no error)"=w121) -> ("New Image"=w117:T5, "error out"=w118:errorcluster)  [unwired: 2 in]
          n44 = call "IMAQ ArrayToImage"("Image Pixels (Float)"=w123, "error in (no error)"=w118, "Image"=w117) -> ("error out"=w122:errorcluster, "Image Out"=w124:T5)  [unwired: 7 in]
          n45 = in-place-cluster #4("Current Dataset Images 1.SGL Image Sum"=w124) -> (w108:T9)
        }
      }
      frame "Mask" {
        n46 = in-place {
          in-place-border: w131 -> [w143]
          in-place-border: [w141] -> w130
          in-place-border: w125 -> [w133]
          in-place-border: w128 -> [w137]
          w134 = T44 7 items=["Grayscale (U8)", "Grayscale (I16)", "Grayscale (SGL)", "Complex (CSG)", "RGB (U32)", "HSL (U32)", "RGB (U64)", "Grayscale (U16)"] ("Image Type")
          n47 = in-place-cluster #5(w127) -> ("Mask Image"=w136:T5)
          n48 = call "Clear Error.vi"("Error In"=w133) -> ("no Error Out"=w132:errorcluster)  [unwired: 8 in]
          n49 = call "IMAQ Dispose"("Image"=w136, "error in (no error)"=w132) -> ("error out"=w139:errorcluster)  [unwired: 4 in]
          n50 = To Unsigned Word Integer(number=w143) -> (unsigned 16bit integer=w140:u16[][])
          n51 = call "IMAQ Create"("Image Name"=w137, "Image Type"=w134, "error in (no error)"=w139) -> ("New Image"=w135:T5, "error out"=w138:errorcluster)  [unwired: 2 in]
          n52 = call "IMAQ ArrayToImage"("Image Pixels (U16)"=w140, "error in (no error)"=w138, "Image"=w135) -> ("error out"=w141:errorcluster, "Image Out"=w142:T5)  [unwired: 7 in]
          n53 = in-place-cluster #5("Mask Image"=w142) -> (w126:T9)
        }
      }
      frame "White Light" {
        n54 = in-place {
          in-place-border: w150 -> [w161]
          in-place-border: [w160] -> w149
          in-place-border: w148 -> [w157]
          in-place-border: w144 -> [w153]
          w156 = T44 7 items=["Grayscale (U8)", "Grayscale (I16)", "Grayscale (SGL)", "Complex (CSG)", "RGB (U32)", "HSL (U32)", "RGB (U64)", "Grayscale (U16)"] ("Image Type")
          n55 = in-place-cluster #6(w146) -> ("White Light Image"=w155:T5)
          n56 = call "Clear Error.vi"("Error In"=w153) -> ("no Error Out"=w151:errorcluster)  [unwired: 8 in]
          n57 = call "IMAQ Dispose"("Image"=w155, "error in (no error)"=w151) -> ("error out"=w159:errorcluster)  [unwired: 4 in]
          n58 = To Unsigned Word Integer(number=w161) -> (unsigned 16bit integer=w152:u16[][])
          n59 = call "IMAQ Create"("Image Name"=w157, "Image Type"=w156, "error in (no error)"=w159) -> ("New Image"=w154:T5, "error out"=w158:errorcluster)  [unwired: 2 in]
          n60 = call "IMAQ ArrayToImage"("Image Pixels (U16)"=w152, "error in (no error)"=w158, "Image"=w154) -> ("error out"=w160:errorcluster, "Image Out"=w162:T5)  [unwired: 7 in]
          n61 = in-place-cluster #6("White Light Image"=w162) -> (w145:T9)
        }
      }
    }
    n62 = in-place-dvr #1(w59) -> (→"Data Value Reference out":refnum<data-value>)  [unwired: 1 out]
  }
  n63 = Format Into String(format string=" plugin:\n%s (%s)", initial string=w5, error in=w56, w6, w39) -> (resulting string=w37:string, error out=w36:errorcluster)
  n64 = Format Into String(format string=" used as %s", initial string=w37, error in=w36, w19) -> (resulting string=→"Message":string, error out=w35:errorcluster)
  n65 = call "Alligator Variables Storage.vi"("Get(F)/Set"=w32, "AlliGator Variable"=w33, "Error In"=w35, "Data in"=w32) -> ("Error Out"=→"error out":errorcluster)  [unwired: 5 in, 2 out]
